vi "setVIName.vi"(8 "error in (no error)":errorcluster, 10 "VI Name":string, 11 "Panel in":refnum<class "Panel.lvclass">) -> (0 "error out":errorcluster, 3 "Panel out":refnum<class "Panel.lvclass">)   [LabVIEW 2019, in "Panel.lvclass"]
uses:
  Panel.lvclass
  Panel.lvclass/Panel.ctl
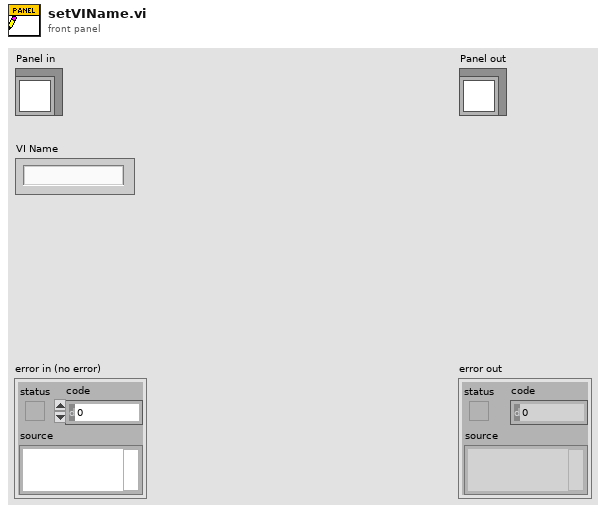
[diagram p1: front panel]
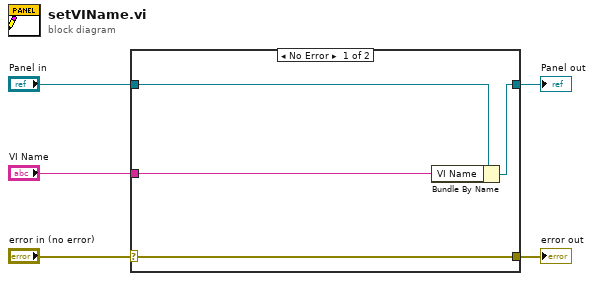
[diagram p0: block diagram]
diagram:
  n1 = case shown="No Error" "error in (no error)" {
    selector: "error in (no error)" -> [w9 w10]
    tunnel: [w9 w10] -> w4
    tunnel: [w7 w11] -> w2
    tunnel: "Panel in" -> [w8 w11]
    tunnel: "VI Name" -> [w6 _]
    frame No Error {
      n2 = Bundle By Name(cluster=w8, "VI Name"=w6) -> (w7:refnum<class "Panel.lvclass">)
    }
    frame Error {
    }
  }
  "error out" <- w4
  "Panel out" <- w2
